vi "Configuration - Get All AI Modules.vi"(11 "Module Configurations":T1[](array[typedef])) -> (1 "AI Found":bool, 2 "AI Modules Configs":T1[](array[typedef]))   [LabVIEW 2017, in "Communications Library.lvlib"]
uses:
  Communications Library.lvlib
  Typedefs/DTACQ Module Configuration--Cluster.ctl
  Typedefs/DTACQ Device Type--Enum.ctl
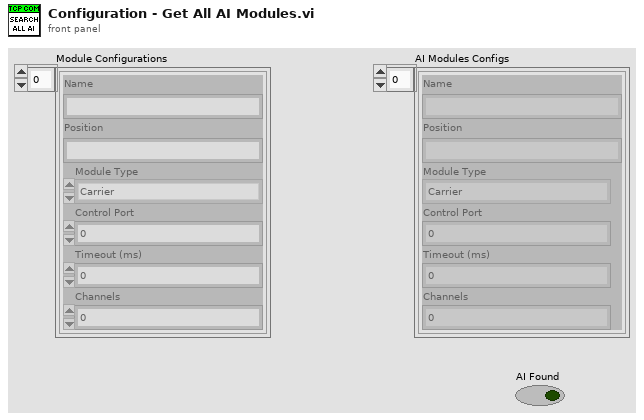
[diagram p1: front panel]
types:
  T1 = typedef "Communications Library.lvlib/DTACQ Module Configuration--Cluster.ctl" = cluster{"Name":string, "Position":string, "Module Type":T2, "Control Port":i32, "Timeout (ms)":i32, "Channels":i32}
  T2 = typedef "Communications Library.lvlib/DTACQ Device Type--Enum.ctl" = enum16{"Carrier", "Analog In Module", "Analog Out Module", "Generic Module"}
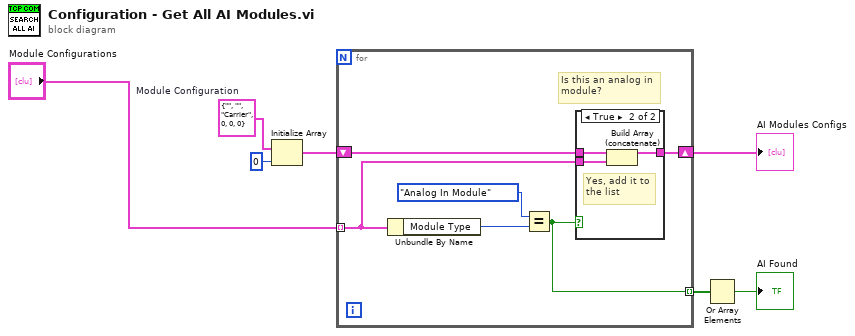
[diagram p0: block diagram]
diagram:
  w6 = T1 {"Name"="", "Position"="", "Module Type"=enum."Carrier", "Control Port"=0, "Timeout (ms)"=0, "Channels"=0}  # Module Configuration
  n1 = Initialize Array(w6, 0 ("dimension size")) -> (w4:T1[])
  n2 = for {
    tunnel: "Module Configurations" -> [w10] mode=indexing
    tunnel: [w8] -> w3 mode=indexing
    shift-right: [w9] -> w1
    shift-left: w4 -> [w11]
    # "Is this an analog in\nmodule?"
    n3 = Unbundle By Name(w10) -> ("Module Type"=w13:T2)
    n4 = Equal?(x=DTACQ_Device_Type--Enum."Analog In Module", y=w13) -> (x = y?=w8:bool)
    n5 = case shown="True" w8 {
      tunnel: w11 -> [w14 w17]
      tunnel: w10 -> [_ w16]
      tunnel: [w14 w15] -> w9
      frame False {
        # "No, do not\nadd it to \nthe list"
      }
      frame True {
        # "Yes, add it to\nthe list"
        n6 = Build Array (concatenate)(w17, w16) -> (w15:T1[])
      }
    }
  }
  "AI Modules Configs" <- w1
  n7 = Or Array Elements(Boolean array=w3) -> (logical OR=→"AI Found":bool)
